vi "Set User Logout.vi"(8 "error in":errorcluster) -> (0 "error out":errorcluster)   [LabVIEW 2012]
doc: "Sets the current user to null."
uses:
  User Access Type defs/User access cluster.ctl
  User Access Type defs/Security level U8.ctl
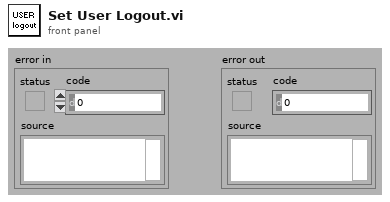
[diagram p1: front panel]
types:
  T1 = typedef "User access cluster.ctl" = cluster{"Active?":bool, "User ID":string, "Password":string, "Name":string, "Security level":T2, "Expired?":bool, "Expire sec":dbl, "Locked?":bool, "New?":bool}
  T2 = typedef "Security level U8.ctl" = u8
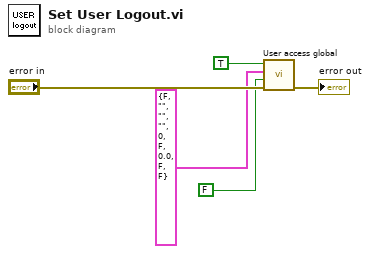
[diagram p0: block diagram]
diagram:
  n1 = call "User access global.vi"("error in (no error)"="error in", "Set Loged in"=FALSE, "User access set"=T1 {"Active?"=FALSE, "User ID"="", "Password"="", "Name"="", "Security level"=0, "Expired?"=FALSE, "Expire sec"=0.0, "Locked?"=FALSE, "New?"=FALSE}, "Set? (get)"=TRUE) -> ("error out"=→"error out":errorcluster)  [unwired: 7 out]
